vi "Get Protection Configuration.vi"(8 "error in":errorcluster, 11 "Parent Ref":T3=18446744073709551615 format="%.0x") -> (0 "error out":errorcluster, 2 "Selected Channels":T1 {"Input Channels"."Node Ref" format="%.0x"}, 3 "Parent Ref Out":T3=18446744073709551615 format="%.0x")   [LabVIEW 2015, in "Protection and Rolling Counter Addon System Explorer.lvlib"]
uses:
  Protection and Rolling Counter Addon System Explorer.lvlib
  <vilib>/NI Veristand/Custom Device API/Custom Device Item Ref.ctl
  Types/Protection Signal Settings.ctl
  Types/Protection Signal Linked Channels.ctl
  Shared/Types/Protection Type.ctl
  Shared/SubVIs/GUID Lookup.vi
  <vilib>/NI Veristand/Custom Device API/Get Item Property (String Array).vi
  <vilib>/NI Veristand/Custom Device API/Get Item Property (Dependent Node Pointer).vi
  <vilib>/NI Veristand/Custom Device API/Get Item Property (U32).vi
  Shared/Protection and Rolling Counter Addon Shared.lvlib
  <vilib>/NI VeriStand/Custom Device API/Custom Device API.lvlib
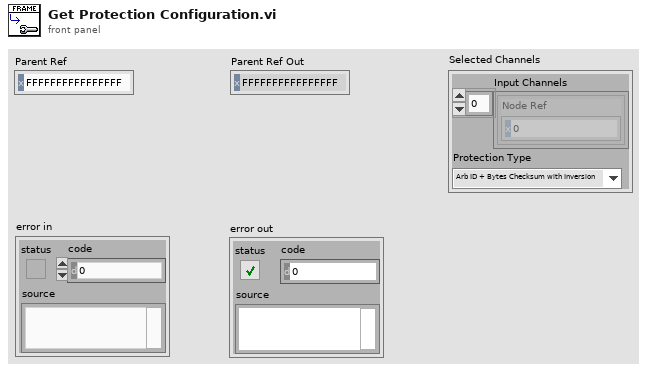
[diagram p1: front panel]
types:
  T1 = typedef "Protection and Rolling Counter Addon System Explorer.lvlib/Protection Signal Settings.ctl" = cluster{"Input Channels":T2[], "Protection Type":T4}
  T2 = typedef "Protection and Rolling Counter Addon System Explorer.lvlib/Protection Signal Linked Channels.ctl" = cluster{"Node Ref":T3}
  T3 = typedef "Custom Device API.lvlib/Custom Device Item Ref.ctl" = u64
  T4 = typedef "Protection and Rolling Counter Addon Shared.lvlib/Protection Type.ctl" = enum16{"Arb ID + Bytes Checksum with Inversion", "Arb ID + Bytes CRC with Inversion", "Reversed Raw Signal Checksum with Inversion"}
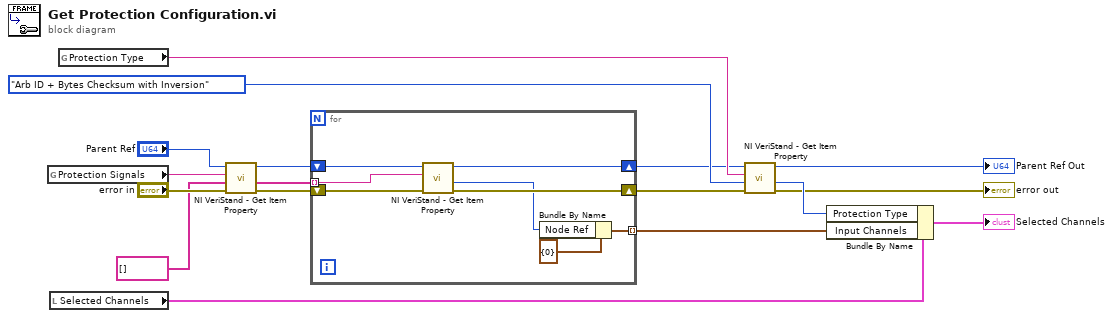
[diagram p0: block diagram]
diagram:
  n1 = global read "GUID Lookup.vi" "Protection Signals"() -> (w15:string)
  n2 = local read "Selected Channels"() -> (w9:T1)
  n3 = global read "GUID Lookup.vi" "Protection Type"() -> (w11:string)
  n4 = call-poly <vilib>:"NI VeriStand - Get Item Property.vi"("error in (no error)"="error in", "Default Value"=string[] [], "Property Name"=w15, "Item Ref in"="Parent Ref") -> ("error out"=w13:errorcluster, "Value"=w6:string[], "Item Ref out"=w12:T3)  [unwired: 4 in, 1 out]
  n5 = for {
    shift-right: [w23] -> w2
    shift-left: w12 -> [w24]
    tunnel: w6 -> [w22] mode=indexing
    shift-right: [w21] -> w5
    shift-left: w13 -> [w25]
    tunnel: [w18] -> w4 mode=indexing
    n6 = call-poly <vilib>:"NI VeriStand - Get Item Property.vi"("error in (no error)"=w25, "Property Name"=w22, "Item Ref in"=w24) -> ("error out"=w21:errorcluster, "Dependent Node Ref"=w19:T3, "Item Ref out"=w23:T3)  [unwired: 5 in, 1 out]
    n7 = Bundle By Name(cluster=T2 {"Node Ref"=0} ("MonitoredChannelSettings"), "Node Ref"=w19) -> (w18:T2)
  }
  n8 = call-poly <vilib>:"NI VeriStand - Get Item Property.vi"("error in (no error)"=w5, "Default Value"=Protection_Type."Arb ID + Bytes Checksum with Inversion" ("Protection Type"), "Property Name"=w11, "Item Ref in"=w2) -> ("error out"=→"error out":errorcluster, "Value"=w8:u32, "Item Ref out"=→"Parent Ref Out":T3)  [unwired: 4 in, 1 out]
  n9 = Bundle By Name(cluster=w9, "Protection Type"=w8, "Input Channels"=w4) -> (→"Selected Channels":T1)
